vi "Parse Synthesizer Data.vi"(8 "error in":errorcluster, 11 "Data":string) -> (0 "error out":errorcluster, 2 "Power":dbl, 3 "Frequency (GHz)":dbl)   [LabVIEW 2019, in "ACSVcontrol-driver.lvlib"]
doc: "Parse data recieved from PJVS with synthesizer data."
uses:
  ACSVcontrol-driver.lvlib
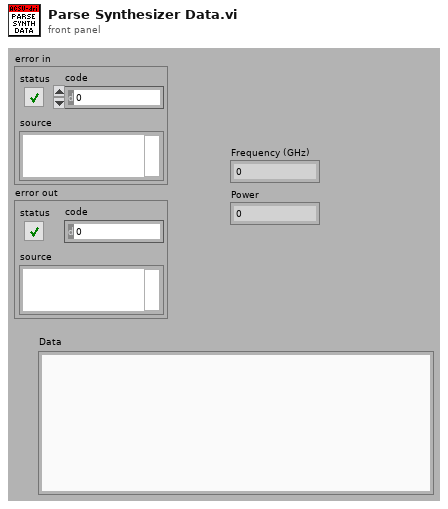
[diagram p1: front panel]
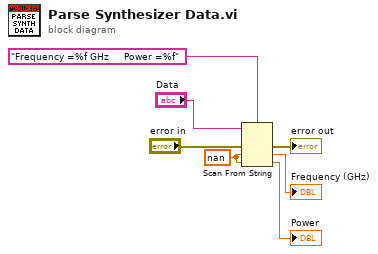
[diagram p0: block diagram]
diagram:
  w3 = nan ("default value 1")
  n1 = Scan From String(format string="Frequency =%f GHz     Power =%f", input string="Data", error in="error in", default 1=w3, default 2=w3) -> (error out=→"error out":errorcluster, output 1=→"Frequency (GHz)":dbl, output 2=→"Power":dbl)  [unwired: 1 in, 2 out]
